vi "Agilent DMM Coerce Range.vi"(9 "Range":T1, 10 "Measurement Type":T2) -> (1 "Coerced Range":T1, 2 "Available Ranges":T1[](array[typedef]))   [LabVIEW 2011]
uses:
  TypeDefs/Agilent DMM Measurement Type.ctl
  TypeDefs/Agilent DMM Range.ctl
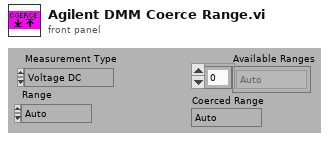
[diagram p1: front panel]
types:
  T1 = typedef "Agilent DMM Range.ctl" = enum16{"Auto", "Min", "Max", "0.01", "0.1", "1", "3", "10", "100", "1,000", "10,000", "100,000", "1,000,000", "10,000,000", "100,000,000"}
  T2 = typedef "Agilent DMM Measurement Type.ctl" = enum16{"Voltage DC", "Voltage DC Ratio", "Voltage AC", "Current DC", "Current AC", "Resistance", "Fresistance", "Frequency", "Period", "Continuity", "Diode"}
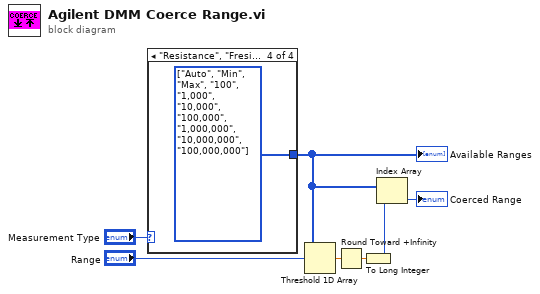
[diagram p0: block diagram]
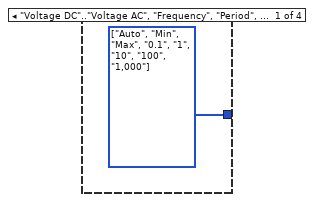
[diagram p2: hidden frame]
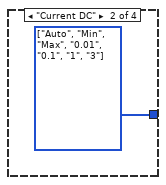
[diagram p3: hidden frame]
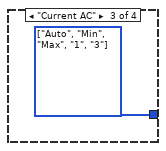
[diagram p4: hidden frame]
diagram:
  n1 = case shown="\"Resistance\", \"Fresistance\"" "Measurement Type" {
    tunnel: [w8 w9 w10 w11] -> w2
    frame "Voltage DC".."Voltage AC", "Frequency", "Period", Default {
      w8 = T1[] [enum."Auto", enum."Min", enum."Max", enum."0.1", enum."1", enum."10", enum."100", enum."1,000"] items=["Auto", "Min", "Max", "0.01", "0.1", "1", "3", "10", "100", "1,000", "10,000", "100,000", "1,000,000", "10,000,000", "100,000,000"]
    }
    frame "Current DC" {
      w9 = T1[] [enum."Auto", enum."Min", enum."Max", enum."0.01", enum."0.1", enum."1", enum."3"] items=["Auto", "Min", "Max", "0.01", "0.1", "1", "3", "10", "100", "1,000", "10,000", "100,000", "1,000,000", "10,000,000", "100,000,000"]
    }
    frame "Current AC" {
      w10 = T1[] [enum."Auto", enum."Min", enum."Max", enum."1", enum."3"] items=["Auto", "Min", "Max", "0.01", "0.1", "1", "3", "10", "100", "1,000", "10,000", "100,000", "1,000,000", "10,000,000", "100,000,000"]
    }
    frame "Resistance", "Fresistance" {
      w11 = T1[] [enum."Auto", enum."Min", enum."Max", enum."100", enum."1,000", enum."10,000", enum."100,000", enum."1,000,000", enum."10,000,000", enum."100,000,000"] items=["Auto", "Min", "Max", "0.01", "0.1", "1", "3", "10", "100", "1,000", "10,000", "100,000", "1,000,000", "10,000,000", "100,000,000"]
    }
  }
  "Available Ranges" <- w2
  n2 = Threshold 1D Array(2:"Range", 3:w2) -> (0:w7:dbl)  [unwired: 1 out]
  n3 = Round Toward +Infinity(x=w7) -> (ceil(x): smallest int >= x=w6:dbl)
  n4 = To Long Integer(number=w6) -> (32bit integer=w3:i32)
  n5 = Index Array(array=w2, index=w3) -> (element=→"Coerced Range":T1)
